vi "编辑控件类型.vi"() -> ()   [LabVIEW 2020]
panel:
  in  "图片路径":path
  in  "修改":bool
  in  "删除":bool
  in  "增加":bool
  in  "控件列表":i32(listbox)
  out "图片预览":picture
  in  "类型名称":string
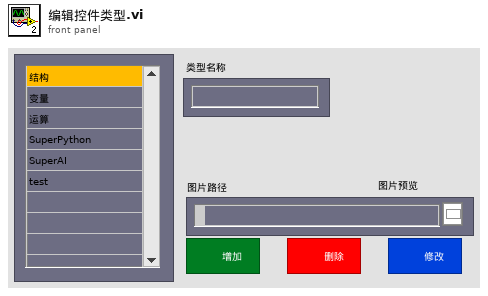
[diagram p1: front panel]
types:
  T1 = typedef "imagedata.ctl" = cluster{"image type":i32, "image depth":i32, "image":u8[], "mask":u8[], "colors":u32[], "Rectangle":cluster{"left":i16, "top":i16, "right":i16, "bottom":i16}}
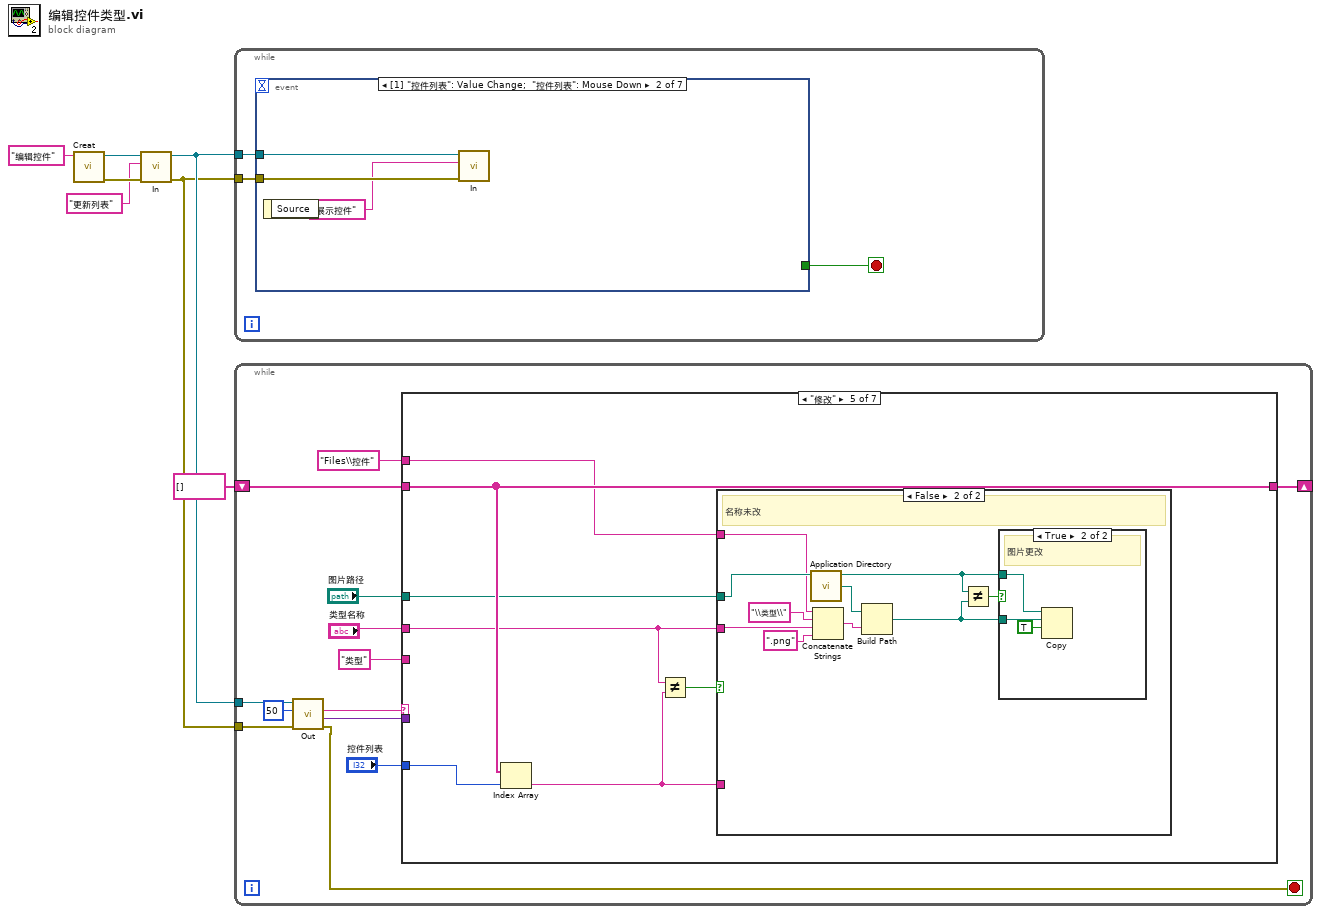
[diagram p0: block diagram]
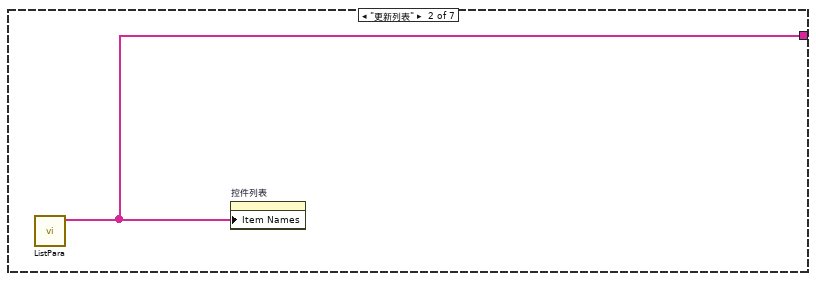
[diagram p3: hidden frame]
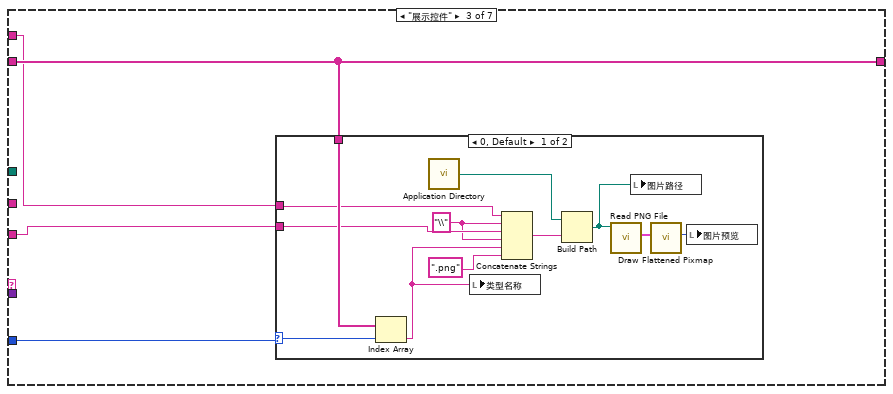
[diagram p4: hidden frame]
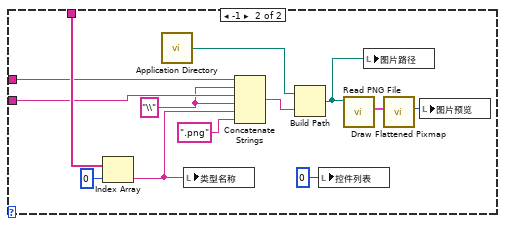
[diagram p5: hidden frame]
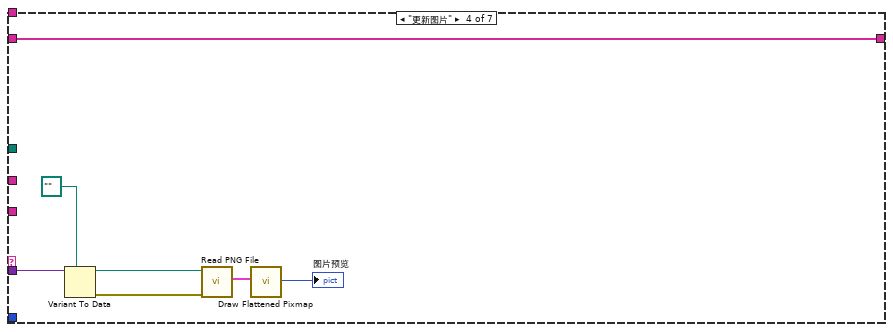
[diagram p6: hidden frame]
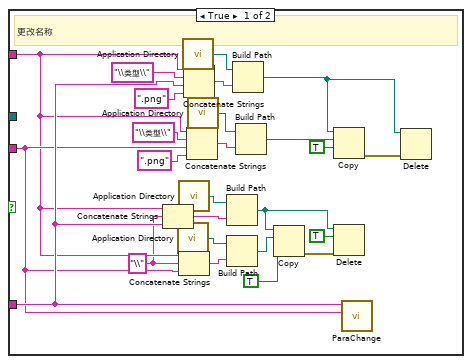
[diagram p7: hidden frame]
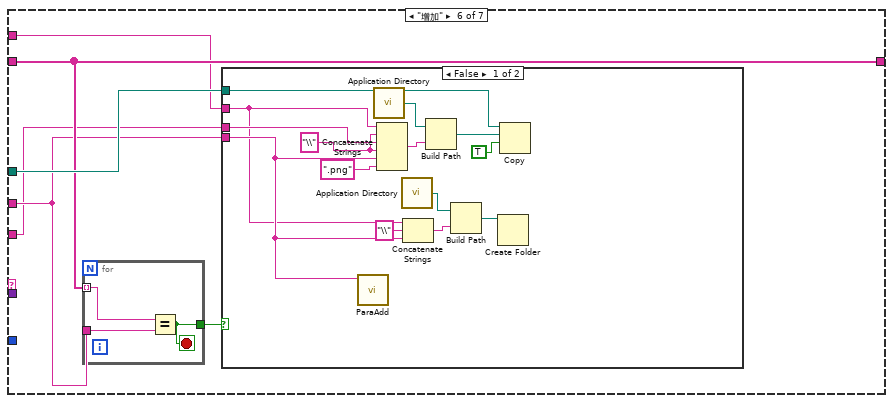
[diagram p9: hidden frame]
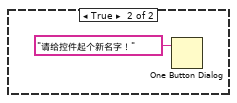
[diagram p10: hidden frame]
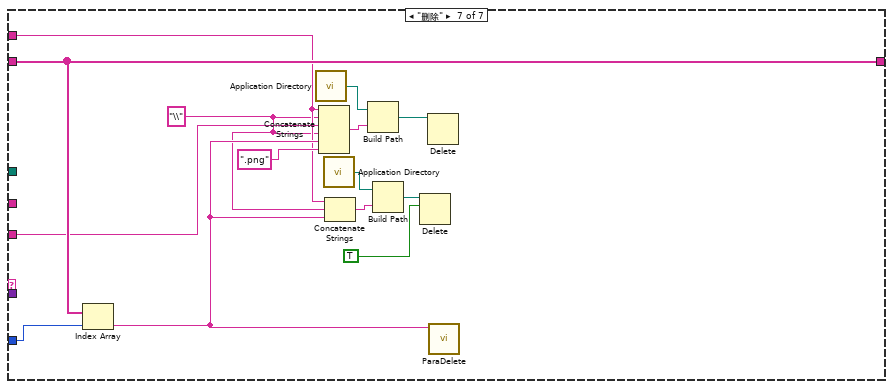
[diagram p11: hidden frame]
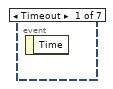
[diagram p12: hidden frame]
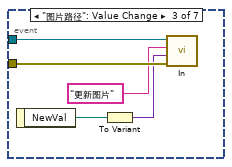
[diagram p13: hidden frame]
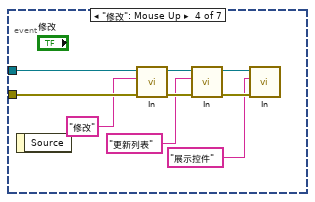
[diagram p14: hidden frame]
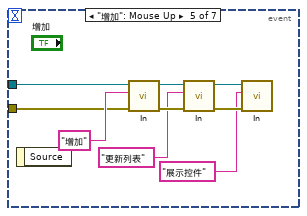
[diagram p15: hidden frame]
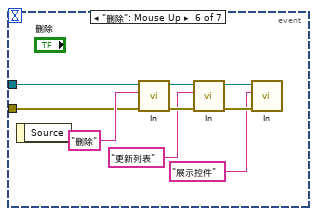
[diagram p16: hidden frame]
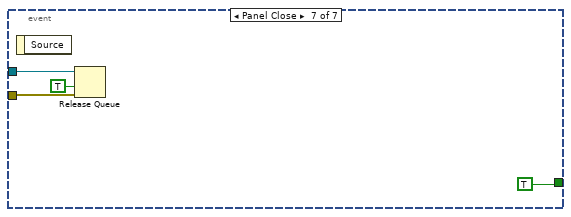
[diagram p17: hidden frame]
diagram:
  n1 = call "Creat.vi"("名称"="编辑控件") -> ("错误输出"=w2:errorcluster, "队列输出"=w5:refnum<queue>)  [unwired: 9 in]
  n2 = call "In.vi"("错误输入"=w2, "指令"="更新列表", "队列"=w5) -> ("错误输出"=w3:errorcluster, "队列输出"=w4:refnum<queue>)  [unwired: 7 in]
  n3 = while {
    tunnel: w4 -> [w10]
    tunnel: w3 -> [w9]
    stop <- w8 stop-if-true
    n4 = event shown="[1] \"控件列表\": Value Change;  \"控件列表\": Mouse Down" {
      selector: _ -> [_ _ _ _ _ _ _]
      dyn-events: _ -> [_ _ _ _ _ _ _]
      timeout: _ -> [_ _ _ _ _ _ _]
      tunnel: w10 -> [_ w13 w18 w27 w29 w38 w48]
      tunnel: w9 -> [_ w12 w17 w26 w28 w37 w47]
      tunnel: [_ _ _ _ _ _ TRUE] -> w8
      event Timeout {
        n5 = event-data() -> ()  [unwired: 1 in, 1 out]
      }
      event "控件列表": Value Change; "控件列表": Mouse Down {
        n6 = event-data() -> ()  [unwired: 1 in, 1 out]
        n7 = call "In.vi"("错误输入"=w12, "指令"="展示控件", "队列"=w13) -> ()  [unwired: 7 in, 2 out]
      }
      event "图片路径": Value Change {
        n8 = event-data() -> ("NewVal"=w16:path)  [unwired: 1 in]
        n9 = To Variant(anything=w16) -> (Variant=w14:variant)
        n10 = call "In.vi"("错误输入"=w17, "数据"=w14, "指令"="更新图片", "队列"=w18) -> ()  [unwired: 6 in, 2 out]
      }
      event "修改": Mouse Up {
        n11 = event-data() -> ()  [unwired: 1 in, 1 out]
        n12 = call "In.vi"("错误输入"=w26, "指令"="修改", "队列"=w27) -> ("错误输出"=w23:errorcluster, "队列输出"=w24:refnum<queue>)  [unwired: 7 in]
        n13 = call "In.vi"("错误输入"=w23, "指令"="更新列表", "队列"=w24) -> ("错误输出"=w21:errorcluster, "队列输出"=w22:refnum<queue>)  [unwired: 7 in]
        n14 = call "In.vi"("错误输入"=w21, "指令"="展示控件", "队列"=w22) -> ()  [unwired: 7 in, 2 out]
      }
      event "增加": Mouse Up {
        n15 = event-data() -> ()  [unwired: 1 in, 1 out]
        n16 = call "In.vi"("错误输入"=w28, "指令"="增加", "队列"=w29) -> ("错误输出"=w34:errorcluster, "队列输出"=w35:refnum<queue>)  [unwired: 7 in]
        n17 = call "In.vi"("错误输入"=w34, "指令"="更新列表", "队列"=w35) -> ("错误输出"=w32:errorcluster, "队列输出"=w33:refnum<queue>)  [unwired: 7 in]
        n18 = call "In.vi"("错误输入"=w32, "指令"="展示控件", "队列"=w33) -> ()  [unwired: 7 in, 2 out]
      }
      event "删除": Mouse Up {
        n19 = event-data() -> ()  [unwired: 1 in, 1 out]
        n20 = call "In.vi"("错误输入"=w37, "指令"="删除", "队列"=w38) -> ("错误输出"=w43:errorcluster, "队列输出"=w44:refnum<queue>)  [unwired: 7 in]
        n21 = call "In.vi"("错误输入"=w43, "指令"="更新列表", "队列"=w44) -> ("错误输出"=w41:errorcluster, "队列输出"=w42:refnum<queue>)  [unwired: 7 in]
        n22 = call "In.vi"("错误输入"=w41, "指令"="展示控件", "队列"=w42) -> ()  [unwired: 7 in, 2 out]
      }
      event Panel Close {
        n23 = event-data() -> ()  [unwired: 1 in, 1 out]
        n24 = Release Queue(queue=w48, force destroy? (F)=TRUE ("强制销毁？(F)"), error in (no error)=w47) -> ()  [unwired: 3 out]
      }
    }
  }
  n25 = while {
    tunnel: w4 -> [w57]
    tunnel: w3 -> [w56]
    shift-right: [w62] -> _
    shift-left: string[] [] ("数据") -> [w61]
    stop <- w53 stop-if-true
    n26 = call "Out.vi"("错误输入"=w56, "超时毫秒(-1)"=50, "队列"=w57) -> ("错误输出"=w53:errorcluster, "数据"=w54:variant, "指令"=w55:string)  [unwired: 5 in, 1 out]
    n27 = case shown="\"修改\"" w55 {
      tunnel: w54 -> [_ _ _ w95 _ _ _]
      tunnel: [w63 w64 w68 w99 w107 w149 w182] -> w62
      tunnel: w61 -> [w63 _ w68 w99 w107 w149 w182]
      tunnel: "类型名称" -> [_ _ _ _ w103 w148 _]
      tunnel: "控件列表" -> [_ _ w67 _ w106 _ w181]
      tunnel: "图片路径" -> [_ _ _ _ w105 w150 _]
      tunnel: "类型" ("字符串") -> [_ _ w66 _ _ w146 w176]
      tunnel: "Files\\控件" ("名称或相对路径") -> [_ _ w65 _ w101 w145 w171]
      frame "null", Default {
      }
      frame "更新列表" {
        n28 = call "ListPara.vi"() -> ("Paras"=w64:string[])  [unwired: 11 in]
        n29 = property on="控件列表" class="LstBox (strict)"("Item Names"=w64) -> ()  [unwired: 2 in, 2 out]
      }
      frame "展示控件" {
        n30 = case shown="0, Default" w67 {
          selector: w67 -> [w72 _]
          tunnel: w68 -> [w73 w87]
          tunnel: w66 -> [w71 w83]
          tunnel: w65 -> [w70 w82]
          frame 0, Default {
            w69 = "\\" ("字符串")
            n31 = Index Array(array=w73, index=w72) -> (element=w74:string)
            n32 = call <vilib>:"Application Directory.vi"() -> ("Application Directory"=w75:path)
            n33 = local write "类型名称"(w74) -> ()
            n34 = Concatenate Strings(w70, w69, w71, w69, w74, ".png" ("字符串")) -> (w76:string)
            n35 = Build Path(base path=w75, name or relative path=w76) -> (appended path=w80:path)
            n36 = call <vilib>:"Read PNG File.vi"("path to PNG file"=w80) -> ("image data"=w78:T1)  [unwired: 8 in, 2 out]
            n37 = local write "图片路径"(w80) -> ()
            n38 = call <vilib>:"Draw Flattened Pixmap.vi"("image data"=w78) -> ("new picture"=w79:picture)  [unwired: 8 in]
            n39 = local write "图片预览"(w79) -> ()
          }
          frame -1 {
            w81 = "\\" ("字符串")
            n40 = Index Array(array=w87, index=0 ("索引")) -> (element=w84:string)
            n41 = call <vilib>:"Application Directory.vi"() -> ("Application Directory"=w88:path)
            n42 = local write "类型名称"(w84) -> ()
            n43 = Concatenate Strings(w82, w81, w83, w81, w84, ".png" ("字符串")) -> (w89:string)
            n44 = Build Path(base path=w88, name or relative path=w89) -> (appended path=w93:path)
            n45 = local write "控件列表"(0 ("控件列表")) -> ()
            n46 = call <vilib>:"Read PNG File.vi"("path to PNG file"=w93) -> ("image data"=w91:T1)  [unwired: 8 in, 2 out]
            n47 = local write "图片路径"(w93) -> ()
            n48 = call <vilib>:"Draw Flattened Pixmap.vi"("image data"=w91) -> ("new picture"=w92:picture)  [unwired: 8 in]
            n49 = local write "图片预览"(w92) -> ()
          }
        }
      }
      frame "更新图片" {
        n50 = Variant To Data(type=path "" ("类型"), Variant=w95) -> (data=w98:path, error out=w94:errorcluster)  [unwired: 1 in]
        n51 = call <vilib>:"Read PNG File.vi"("error in (no error)"=w94, "path to PNG file"=w98) -> ("image data"=w100:T1)  [unwired: 7 in, 2 out]
        n52 = call <vilib>:"Draw Flattened Pixmap.vi"("image data"=w100) -> ("new picture"=→"图片预览":picture)  [unwired: 8 in]
      }
      frame "修改" {
        n53 = Index Array(array=w107, index=w106) -> (element=w102:string)
        n54 = Not Equal?(x=w103, y=w102) -> (x != y?=w104:bool)
        n55 = case shown="False" w104 {
          tunnel: w105 -> [_ w135]
          tunnel: w102 -> [w112 _]
          tunnel: w103 -> [w111 w137]
          tunnel: w101 -> [w110 w133]
          frame True {
            w109 = "\\" ("字符串")
            # "更改名称"
            n56 = Concatenate Strings(w110, w109, w112) -> (w125:string)
            n57 = call <vilib>:"Application Directory.vi"() -> ("Application Directory"=w123:path)
            n58 = call <vilib>:"Application Directory.vi"() -> ("Application Directory"=w126:path)
            n59 = Concatenate Strings(w110, w109, w111) -> (w124:string)
            n60 = call <vilib>:"Application Directory.vi"() -> ("Application Directory"=w115:path)
            n61 = Concatenate Strings(w110, "\\类型\\" ("名称或相对路径"), w112, ".png" ("字符串")) -> (w116:string)
            n62 = Concatenate Strings(w110, "\\类型\\" ("名称或相对路径"), w111, ".png" ("字符串")) -> (w130:string)
            n63 = call <vilib>:"Application Directory.vi"() -> ("Application Directory"=w129:path)
            n64 = Build Path(base path=w126, name or relative path=w125) -> (appended path=w121:path)
            n65 = Build Path(base path=w123, name or relative path=w124) -> (appended path=w122:path)
            n66 = Build Path(base path=w115, name or relative path=w116) -> (appended path=w114:path)
            n67 = Build Path(base path=w129, name or relative path=w130) -> (appended path=w131:path)
            n68 = Copy(9:TRUE ("覆盖(F)"), 10:w122, 11:w121) -> (0:w120:errorcluster)  [unwired: 2 in, 2 out]
            n69 = Copy(9:TRUE ("覆盖(F)"), 10:w131, 11:w114) -> (0:w119:errorcluster)  [unwired: 2 in, 2 out]
            n70 = Delete(path (use dialog)=w121, entire hierarchy (F)=TRUE ("整个层次结构(F)"), error in=w120) -> ()  [unwired: 2 in, 3 out]
            n71 = call "ParaChange.vi"("新段名"=w111, "原段名"=w112) -> ()  [unwired: 10 in]
            n72 = Delete(path (use dialog)=w114, error in=w119) -> ()  [unwired: 3 in, 3 out]
          }
          frame False {
            # "名称未改"
            n73 = call <vilib>:"Application Directory.vi"() -> ("Application Directory"=w140:path)
            n74 = Concatenate Strings(w133, "\\类型\\" ("名称或相对路径"), w137, ".png" ("字符串")) -> (w141:string)
            n75 = Build Path(base path=w140, name or relative path=w141) -> (appended path=w134:path)
            n76 = Not Equal?(x=w135, y=w134) -> (x != y?=w136:bool)
            n77 = case shown="True" w136 {
              tunnel: w134 -> [_ w143]
              tunnel: w135 -> [_ w142]
              frame False {
                # "图片未改"
              }
              frame True {
                # "图片更改"
                n78 = Copy(9:TRUE ("覆盖(F)"), 10:w143, 11:w142) -> ()  [unwired: 2 in, 3 out]
              }
            }
          }
        }
      }
      frame "增加" {
        n79 = for {
          tunnel: w149 -> [w151] mode=indexing
          tunnel: w148 -> [w153]
          tunnel: [w152] -> w147
          stop <- w152 stop-if-true
          n80 = Equal?(x=w151, y=w153) -> (x = y?=w152:bool)
        }
        n81 = case shown="False" w147 {
          tunnel: w148 -> [w159 _]
          tunnel: w150 -> [w164 _]
          tunnel: w146 -> [w162 _]
          tunnel: w145 -> [w156 _]
          frame False {
            w155 = "\\" ("字符串")
            n82 = call "ParaAdd.vi"("段名"=w159) -> ()  [unwired: 11 in]
            n83 = call <vilib>:"Application Directory.vi"() -> ("Application Directory"=w166:path)
            n84 = Concatenate Strings(w156, w155, w162, w155, w159, ".png" ("字符串")) -> (w167:string)
            n85 = call <vilib>:"Application Directory.vi"() -> ("Application Directory"=w160:path)
            n86 = Concatenate Strings(w156, "\\" ("字符串"), w159) -> (w158:string)
            n87 = Build Path(base path=w166, name or relative path=w167) -> (appended path=w161:path)
            n88 = Build Path(base path=w160, name or relative path=w158) -> (appended path=w157:path)
            n89 = Create Folder(path (use dialog)=w157) -> ()  [unwired: 2 in, 3 out]
            n90 = Copy(9:TRUE ("覆盖(F)"), 10:w161, 11:w164) -> ()  [unwired: 2 in, 3 out]
          }
          frame True {
            n91 = One Button Dialog(message="请给控件起个新名字！" ("消息")) -> ()  [unwired: 1 in, 1 out]
          }
        }
      }
      frame "删除" {
        w170 = "\\" ("字符串")
        n92 = Index Array(array=w182, index=w181) -> (element=w172:string)
        n93 = call <vilib>:"Application Directory.vi"() -> ("Application Directory"=w179:path)
        n94 = Concatenate Strings(w171, w170, w176, w170, w172, ".png" ("字符串")) -> (w180:string)
        n95 = call <vilib>:"Application Directory.vi"() -> ("Application Directory"=w175:path)
        n96 = Concatenate Strings(w171, w170, w172) -> (w174:string)
        n97 = Build Path(base path=w179, name or relative path=w180) -> (appended path=w177:path)
        n98 = Build Path(base path=w175, name or relative path=w174) -> (appended path=w173:path)
        n99 = Delete(path (use dialog)=w173, entire hierarchy (F)=TRUE ("整个层次结构(F)")) -> ()  [unwired: 3 in, 3 out]
        n100 = Delete(path (use dialog)=w177) -> ()  [unwired: 4 in, 3 out]
        n101 = call "ParaDelete.vi"("段名"=w172) -> ()  [unwired: 11 in]
      }
    }
  }
